vi "Build Report String.vi"(8 "error in (no error)":errorcluster, 10 "Report Data":T1, 11 "Macro Step in":refnum<class "Macro Step.lvclass">) -> (0 "error out":errorcluster, 2 "Report String":string, 3 "Macro Step out":refnum<class "Macro Step.lvclass">)   [LabVIEW 2020, in "MacroAssert.lvlib" / "Macro Step.lvclass"]
doc: "Builds a string using <B>Step</B> and <B>Report Data</B> to be included in a report."
uses:
  Macro Step.lvclass
  Macro Step.lvclass/Macro Step.ctl
  Step/Step.lvclass
  CTLs/Report Data.ctl
  MacroAssert.lvlib
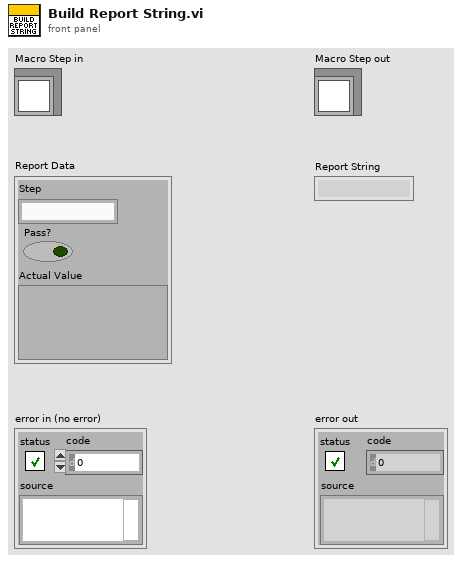
[diagram p1: front panel]
types:
  T1 = typedef "MacroAssert.lvlib/Report Data.ctl" = cluster{"Step":string, "Pass?":bool, "Actual Value":variant}
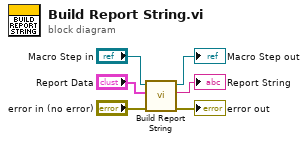
[diagram p0: block diagram]
diagram:
  n1 = call-parent "Build Report String.vi"("error in (no error)"="error in (no error)", "Report Data"="Report Data", "Step in"="Macro Step in") -> ("error out"=→"error out":errorcluster, "Report String"=→"Report String":string, "Step out"=→"Macro Step out":refnum<class "Macro Step.lvclass">)  [unwired: 6 in]
